vi "Host.vi"() -> ()   [LabVIEW 2017]
uses:
  <vilib>/NI/STM/TCP/TCP Read Options.ctl
  TypeDefs/Data for Logging.ctl
  TypeDefs/ClientStatusData.ctl
  <vilib>/NI/STM/TCP/Read Meta Data (TCP Ref).vi
  <vilib>/NI/STM/TCP/Get Connection Reference (TCP).vi
  <vilib>/NI/STM/TCP/Read Meta Data (TCP Clst).vi
  <vilib>/NI/STM/TCP/Write Message (TCP).vi
  <vilib>/NI/STM/TCP/Read Message (TCP).vi
  <vilib>/NI/STM/NI STM.lvlib
panel:
  out "Numeric 2":dbl
  out "Numeric":dbl
  in  "C":dbl=1.0
  in  "K":dbl=1.0
  in  "D":dbl
  in  "I":dbl
  in  "P":dbl=0.2
  in  "Update":bool
  in  "testingtargetY":dbl=0.1
  in  "testingtargetX":dbl=0.1
  in  "Testing?":bool
  out "RECENT PLAYERS":string[](array[string])
  out "X POSITION":cluster{dbl, dbl}(graph)
  out "Y POSITION":cluster{dbl, dbl}(graph)
  out "?":cluster{dbl[], dbl[]}[](graph)
  in  "assistance":bool
  out "error  out":errorcluster
  in  "stop":bool
  # "zero gains here create NaN (bad for controller)"
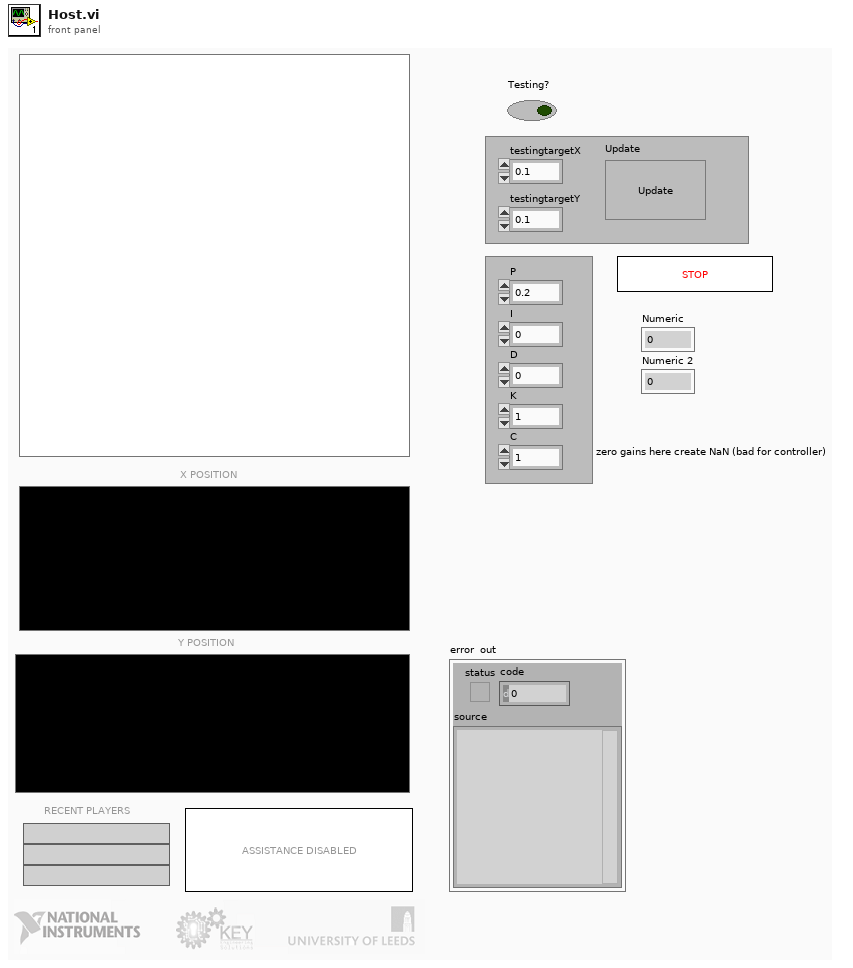
[diagram p1: front panel]
types:
  T1 = typedef "NI STM.lvlib/TCP Connection Info.ctl" = cluster{"connection ID":refnum<k5>, "meta data":T2[]}
  T2 = typedef "NI STM.lvlib/MetaDataElement.ctl" = string
  T3 = typedef "NI STM.lvlib/TCP Read Options.ctl" = cluster{"ignore timeout error":bool, "timeout ms (1000)":i32}
  T4 = enum16{"open", "replace", "create", "open or create", "replace or create", "replace or create with confirmation"}
  T5 = typedef "Data for Logging.ctl" = cluster{"end effector x (mm)":dbl, "end effector y (mm)":dbl, "target x (mm)":dbl, "target y (mm)":dbl, "Theta 1":dbl, "Theta 2":dbl, "Omega 1":dbl, "Omega 2":dbl}
  T6 = typedef "ClientStatusData.ctl" = cluster{"gameState":u16, "playerName":string, "playerScore":dbl, "gameUnits":string}
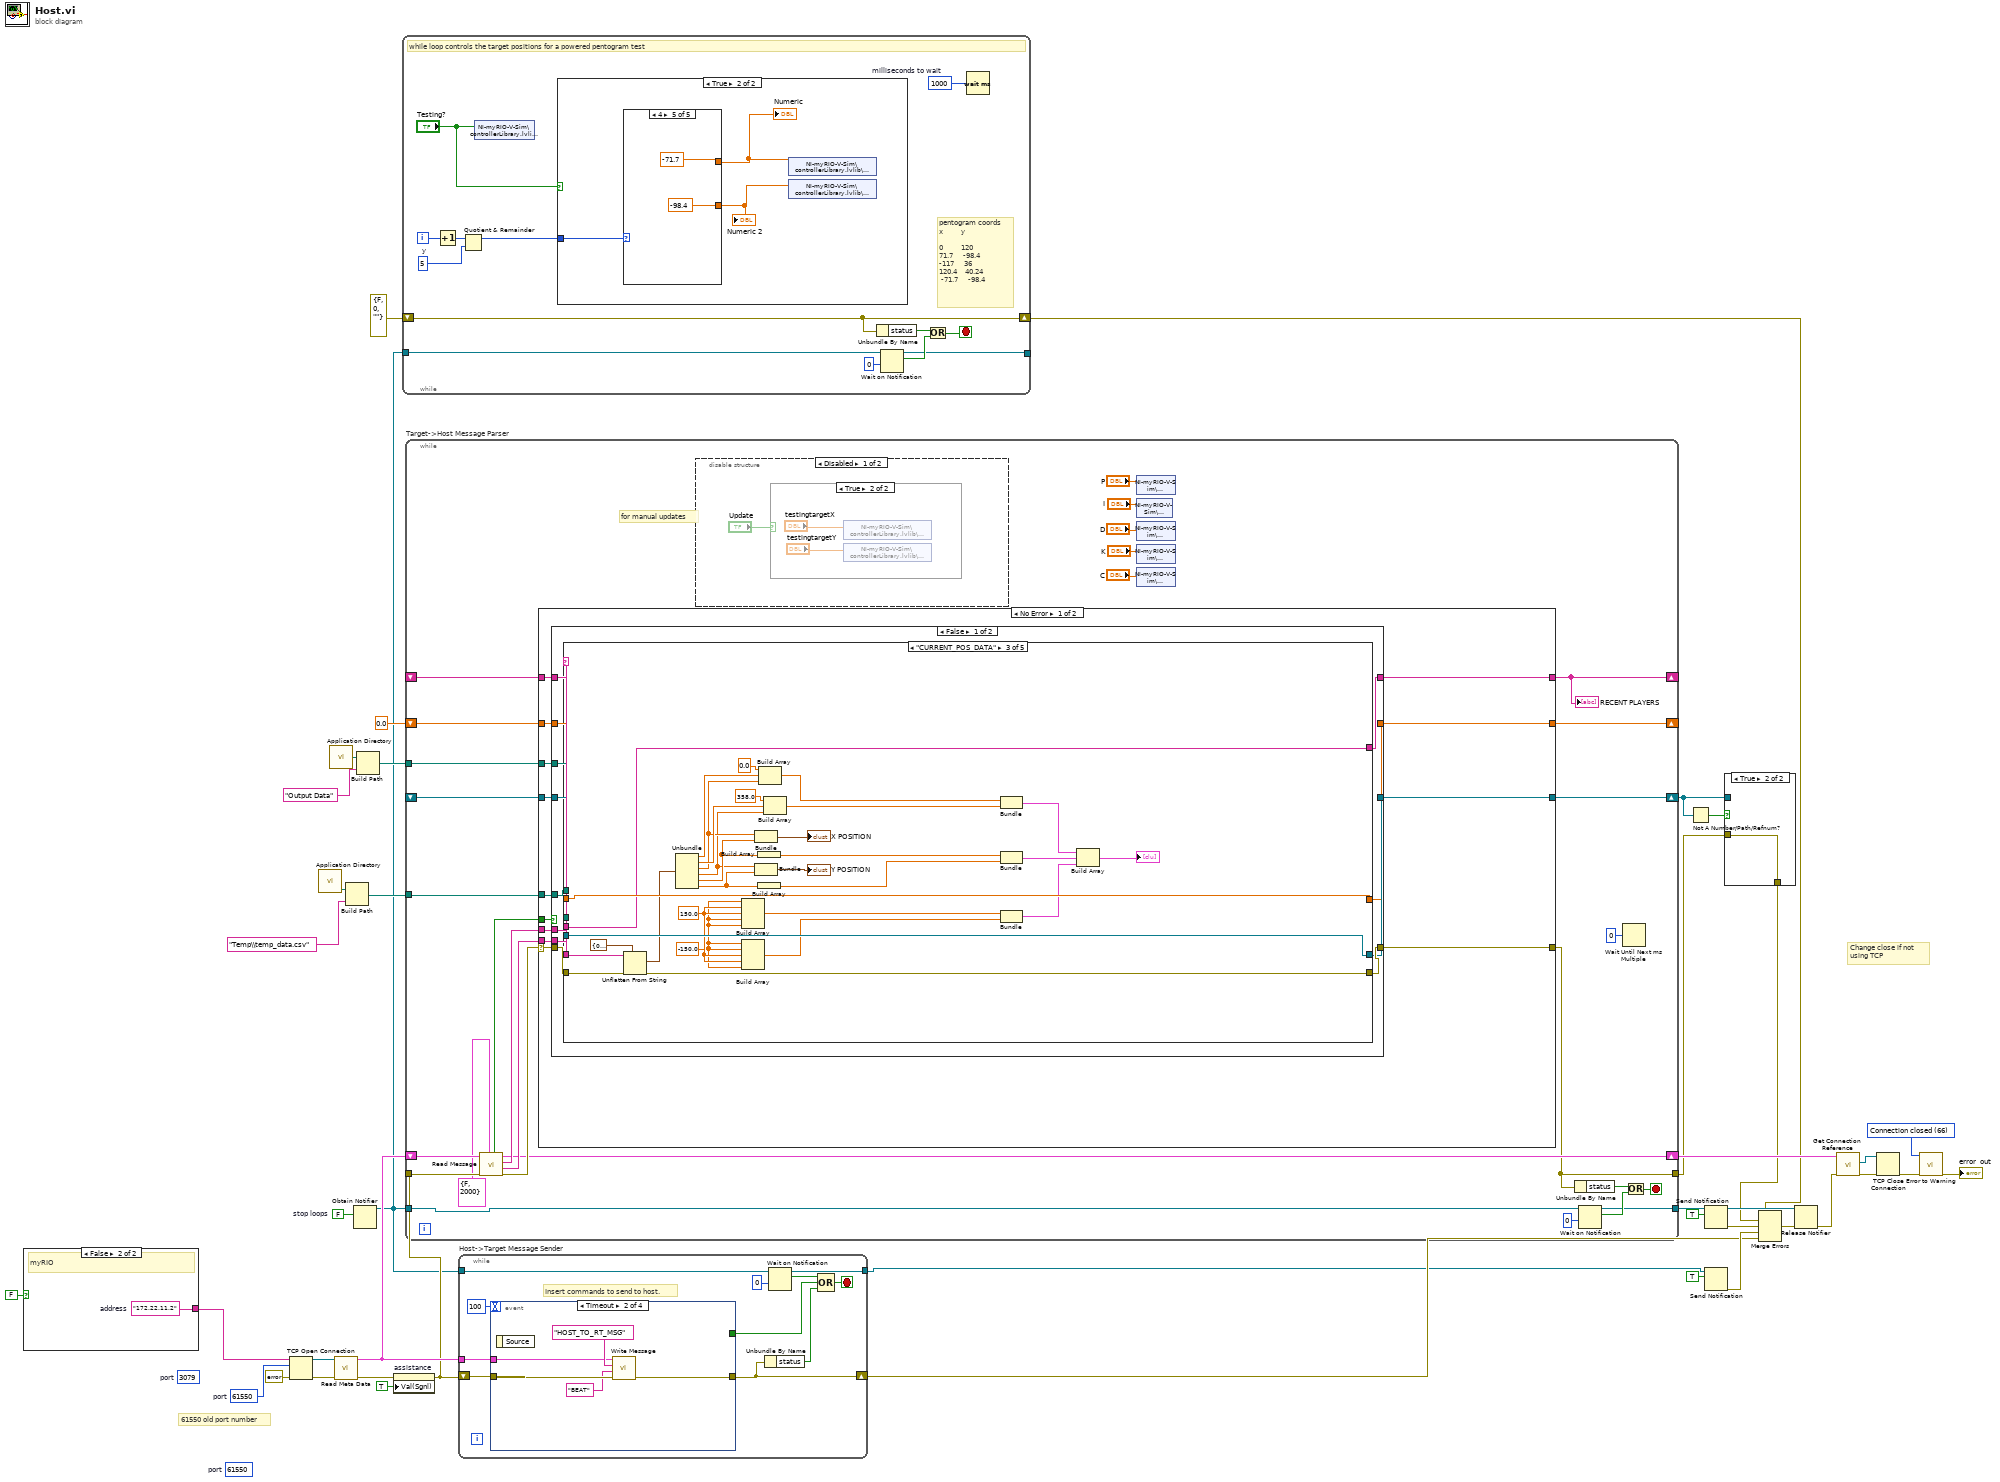
[diagram p0: block diagram]
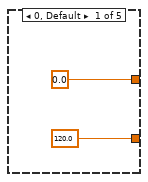
[diagram p3: hidden frame]
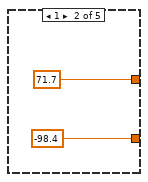
[diagram p4: hidden frame]
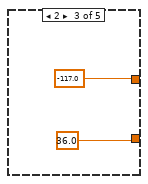
[diagram p5: hidden frame]
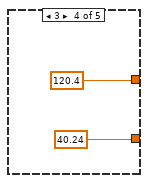
[diagram p6: hidden frame]
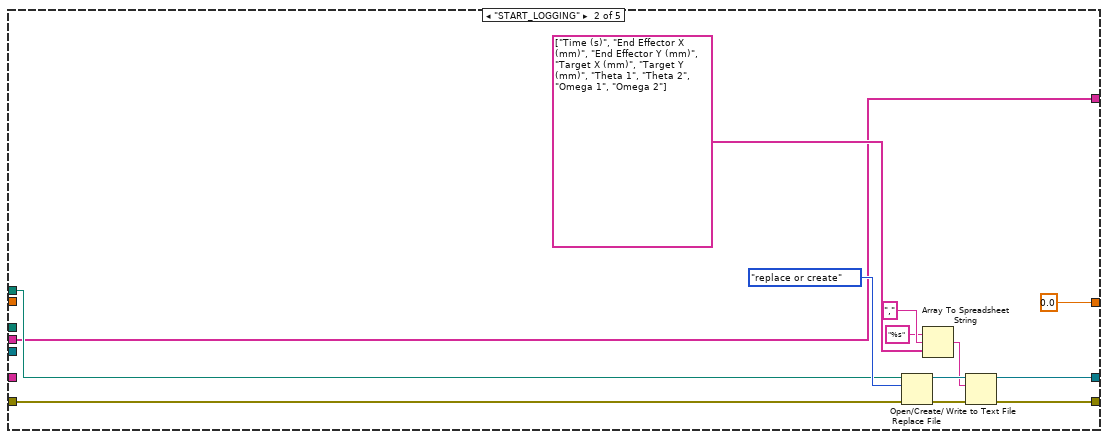
[diagram p10: hidden frame]
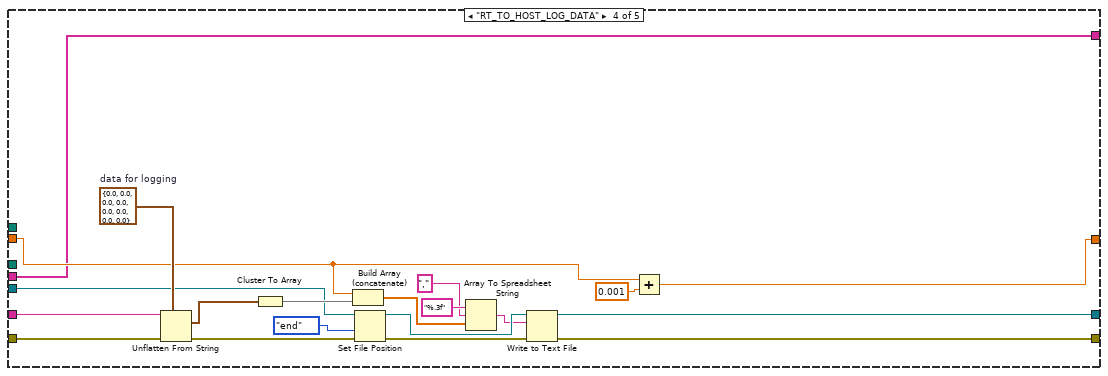
[diagram p11: hidden frame]
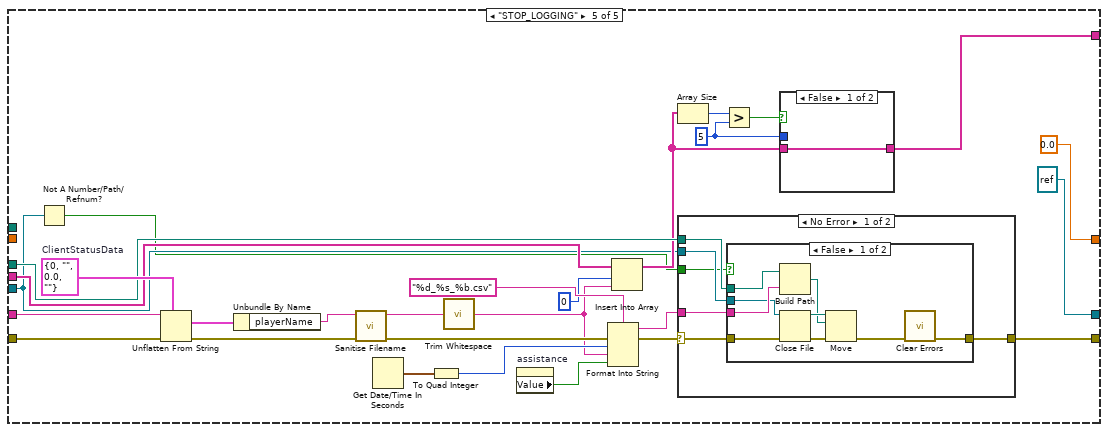
[diagram p12: hidden frame]
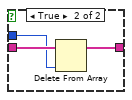
[diagram p15: hidden frame]
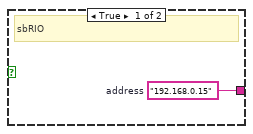
[diagram p18: hidden frame]
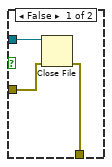
[diagram p19: hidden frame]
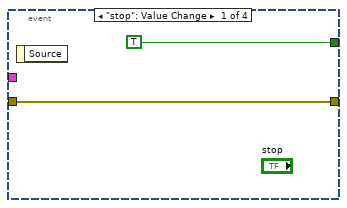
[diagram p20: hidden frame]
diagram:
  (unwired) u16 61550  # port
  w5 = u16 61550  # port
  w26 = FALSE  # stop loops
  w37 = 66 items=["No Error", "Argument Error", "Memory Full", "Out of Zone", "End of File", "File Already Open", "Generic File IO Error", "File Not Found", "File Permission Error", "Disk Full", "Duplicate Path", "Too Many Files Open", "Not Enabled", "Resource File Not Found", "Cannot Add Resource", "Resource Not Found", "Image Not Found", "Image Memory Error", "Pen Does Not Exist", "Config Bad Type", "Config Token Not Found", "Config Parse Error", "Config Memory Error", "Bad External Code Format", "Bad External Code Offset", "External Code Not Present", "Null Window", "Destroy Window Mixup", "Null Menu", "Print Aborted", "Bad Print Record", "Print Driver Error", "Windows Error During Print", "Memory Error During Print", "Print Dialog Error", "Generic Print Error", "Invalid Device Refnum", "Device Not Found", "Device Parameter Error", "Device Unit Error", "Can't Open Device", "Device Call Aborted", "Generic Error", "Cancelled By User", "Object ID Too Low", "Object ID Too High", "Object Not In Heap", "Unknown Heap", "Bad DefProc ID", "DefProc Not In Table", "Message Out Of Range", "Null Method", "Unknown Message", "Manager Call Not Supported", "Bad address", "Connection In progress", "Connection timed out", "Connection is already in progress", "Network attribute not supported", "Network error", "Address in use", "System out of memory", "Connection aborted", "Connection refused", "Connection is not connected", "Connection is already connected", "Connection closed", "Initialize error (interapplication manager)", "Bad occurrence", "Wait on unbound occurrence handler", "Occurrence queue overflow", "Bad path", "Semaphore not signaled", "Unrecognized type (interapplication manager)"] ("1st Error to Convert")
  (unwired) u16 3079  # port
  # "61550 old port number"
  # "Change close if not using TCP"
  n1 = case shown="False" FALSE {
    tunnel: [w42 w43] -> w41
    frame True {
      w42 = "192.168.0.15"  # address
      # "sbRIO"
    }
    frame False {
      w43 = "172.22.11.2"  # address
      # "myRIO"
    }
  }
  n2 = TCP Open Connection(address=w41, remote port or service name=w5, error in (no error)=errorcluster {"status"=FALSE, "code"=0, "source"=""}) -> (connection ID=w21:refnum<k5>, error out=w20:errorcluster)  [unwired: 2 in]
  n3 = call <vilib>:"Application Directory.vi"() -> ("Application Directory"=w18:path)
  n4 = call <vilib>:"Application Directory.vi"() -> ("Application Directory"=w16:path)
  n5 = call-poly <vilib>:"Read Meta Data.vi"("error in"=w20, "connection ID"=w21) -> ("error out"=w11:errorcluster, "connection info out"=w24:T1)  [unwired: 1 in, 7 out]
  n6 = Build Path(base path=w18, name or relative path="Temp\\temp_data.csv") -> (appended path=w17:path)
  n7 = Obtain Notifier(notification data type=w26) -> (notifier out=w3:refnum<notifier>)  [unwired: 3 in, 2 out]
  n8 = Build Path(base path=w16, name or relative path="Output Data") -> (appended path=w14:path)
  n9 = property on="assistance" class="Bool (strict)"(error in=w11, "Val(Sgnl)"=TRUE ("Value (Signaling)")) -> (error out=w10:errorcluster)  [unwired: 1 in, 1 out]
  n10 = while {
    tunnel: w3 -> [w53]
    tunnel: [w52] -> _
    shift-right: [w50] -> w1
    shift-left: errorcluster {"status"=FALSE, "code"=0, "source"=""} ("error constant") -> [w50]
    i -> [w47]
    stop <- w51 stop-if-true
    w45 = 5  # y
    w48 = u32 1000  # milliseconds to wait
    # "pentogram coords\nx         y \n\n0         120\n71.7     -98.4\n-117     36\n120.4    40.24 \n -71.7     -98.4"
    # "while loop controls the target positions for a powered pentogram test"
    n11 = Increment(x=w47) -> (x+1=w46:i32)
    n12 = Quotient & Remainder(x=w46, y=w45) -> (x-y*floor(x/y)=w44:i32)  [unwired: 1 out]
    n13 = shared-variable "NI-myRIO-V-Sim\\controllerLibrary.lvlib\\testing"("Testing?") -> ()  [unwired: 1 in, 1 out]
    n14 = case shown="True" "Testing?" {
      tunnel: w44 -> [_ w59]
      frame False {
      }
      frame True {
        n15 = case shown="4" w59 {
          tunnel: [0.0 71.7 -117.0 120.4 -71.7] -> w58
          tunnel: [120.0 -98.4 36.0 40.24 -98.4] -> w57
          frame 0, Default {
          }
          frame 1 {
          }
          frame 2 {
          }
          frame 3 {
          }
          frame 4 {
          }
        }
        "Numeric" <- w58
        "Numeric 2" <- w57
        n16 = shared-variable "NI-myRIO-V-Sim\\controllerLibrary.lvlib\\testingtargetX"(w58) -> ()  [unwired: 1 in, 1 out]
        n17 = shared-variable "NI-myRIO-V-Sim\\controllerLibrary.lvlib\\testingtargetY"(w57) -> ()  [unwired: 1 in, 1 out]
      }
    }
    n18 = Unbundle By Name(w50) -> ("status"=w54:bool)
    n19 = Wait on Notification(notifier=w53, timeout in ms (-1)=0) -> (notifier out=w52:refnum<notifier>, notification=w55:bool)  [unwired: 2 in, 2 out]
    n20 = Or(x=w54, y=w55) -> (x .or. y?=w51:bool)
    n21 = Wait (ms)(milliseconds to wait=w48) -> ()  [unwired: 1 out]
  }
  n22 = while "Target->Host Message Parser" {
    tunnel: w3 -> [w91]
    tunnel: [w87] -> w27
    shift-right: [w92] -> w25
    shift-left: w24 -> [w98]
    tunnel: w17 -> [w83]
    tunnel: w14 -> [w82]
    shift-right: [w81] -> w8
    shift-left: _ -> [w80]
    shift-right: [w78] -> _
    shift-left: 0.0 -> [w79]
    shift-right: [w76] -> _
    shift-left: _ -> [w77]
    tunnel: w10 -> [w97]
    tunnel: [w85] -> w4
    stop <- w88 stop-if-true
    # "for manual updates"
    n23 = call-poly <vilib>:"Read Message.vi"("options"=T3 {"ignore timeout error"=FALSE, "timeout ms (1000)"=2000}, "error in"=w97, "connection info in"=w98) -> ("error out"=w93:errorcluster, "name"=w96:T2, "data string"=w95:string, "connection info out"=w92:T1, "timed out?"=w94:bool)  [unwired: 2 in, 2 out]
    n24 = case shown="No Error" w93 {
      selector: w93 -> [w111 w250]
      tunnel: w96 -> [w114 _]
      tunnel: w95 -> [w113 _]
      tunnel: w94 -> [w112 _]
      tunnel: [w110 w250] -> w85
      tunnel: w83 -> [w109 _]
      tunnel: w82 -> [w108 _]
      tunnel: [w107 w249] -> w81
      tunnel: w80 -> [w106 w249]
      tunnel: w79 -> [w105 w248]
      tunnel: [w104 w248] -> w78
      tunnel: w77 -> [w103 w247]
      tunnel: [w102 w247] -> w76
      frame No Error {
        n25 = case shown="False" w112 {
          tunnel: w114 -> [w123 _]
          tunnel: w113 -> [w126 _]
          tunnel: w111 -> [w125 w246]
          tunnel: [w124 w246] -> w110
          tunnel: w109 -> [w122 _]
          tunnel: w108 -> [w121 _]
          tunnel: [w120 w245] -> w107
          tunnel: w106 -> [w119 w245]
          tunnel: w105 -> [w118 w244]
          tunnel: [w117 w244] -> w104
          tunnel: w103 -> [w116 w243]
          tunnel: [w115 w243] -> w102
          frame False {
            n26 = case shown="\"CURRENT_POS_DATA\"" w123 {
              tunnel: w126 -> [_ _ w170 w191 w219]
              tunnel: w125 -> [w128 w142 w169 w193 w221]
              tunnel: [w128 w139 w168 w177 w195] -> w124
              tunnel: w122 -> [_ w141 _ _ _]
              tunnel: w121 -> [_ _ _ _ w213]
              tunnel: [w130 w138 w172 w176 refnum<file> refnum ("refnum out")] -> w120
              tunnel: w119 -> [w130 _ w172 w175 w197]
              tunnel: w118 -> [w129 _ w173 w186 _]
              tunnel: [w129 0.0 w173 w188 0.0] -> w117
              tunnel: w116 -> [w127 w131 w147 w174 w205]
              tunnel: [w127 w131 w147 w174 w200] -> w115
              frame Default {
              }
              frame "START_LOGGING" {
                n27 = Open/Create/Replace File(file path (use dialog)=w141, error in=w142, operation (0:open)=T4."replace or create") -> (refnum out=w134:refnum<file>, error out=w135:errorcluster)  [unwired: 3 in, 1 out]
                n28 = Array To Spreadsheet String(delimiter (Tab)=",", array=string[] ["Time (s)", "End Effector X (mm)", "End Effector Y (mm)", "Target X (mm)", "Target Y (mm)", "Theta 1", "Theta 2", "Omega 1", "Omega 2"], 3:"%s" ("format string")) -> (spreadsheet string=w133:string)
                n29 = Write to Text File(file (use dialog)=w134, text=w133, error in=w135) -> (refnum out=w138:refnum<file>, error out=w139:errorcluster)  [unwired: 1 in, 1 out]
              }
              frame "CURRENT_POS_DATA" {
                w152 = -150.0
                w153 = 150.0
                n30 = Unflatten From String(type=cluster{dbl, dbl, dbl, dbl, dbl, dbl} {0.0, 0.0, 0.0, 0.0, 0.0, 0.0}, binary string=w170, error in (no error)=w169) -> (value=w167:cluster{dbl, dbl, dbl, dbl, dbl, dbl}, error out=w168:errorcluster)  [unwired: 2 in, 1 out]
                n31 = Unbundle(w167) -> (w164:dbl, w163:dbl, w145:dbl, w144:dbl, w150:dbl, w151:dbl)
                n32 = Build Array(w152, w153, w153, w152, w152) -> (w155:dbl[])
                n33 = Build Array(w152, w152, w153, w153, w152) -> (w154:dbl[])
                n34 = Bundle(w145, w150) -> (→"X POSITION":cluster{dbl, dbl})  [unwired: 1 in]
                n35 = Bundle(w144, w151) -> (→"Y POSITION":cluster{dbl, dbl})  [unwired: 1 in]
                n36 = Build Array(w150) -> (w158:dbl[])
                n37 = Build Array(w151) -> (w157:dbl[])
                n38 = Build Array(0.0 ("element"), w164, w145) -> (w162:dbl[])
                n39 = Build Array(358.0 ("element"), w163, w144) -> (w161:dbl[])
                n40 = Bundle(w162, w161) -> (w160:cluster{dbl[], dbl[]})  [unwired: 1 in]
                n41 = Bundle(w158, w157) -> (w156:cluster{dbl[], dbl[]})  [unwired: 1 in]
                n42 = Bundle(w155, w154) -> (w146:cluster{dbl[], dbl[]})  [unwired: 1 in]
                n43 = Build Array(w160, w156, w146) -> (→"?":cluster{dbl[], dbl[]}[])
              }
              frame "RT_TO_HOST_LOG_DATA" {
                w192 = T5 {"end effector x (mm)"=0.0, "end effector y (mm)"=0.0, "target x (mm)"=0.0, "target y (mm)"=0.0, "Theta 1"=0.0, "Theta 2"=0.0, "Omega 1"=0.0, "Omega 2"=0.0}  # data for logging
                n44 = Unflatten From String(type=w192, binary string=w191, error in (no error)=w193) -> (value=w190:T5, error out=w182:errorcluster)  [unwired: 2 in, 1 out]
                n45 = Cluster To Array(cluster=w190) -> (array=w187:dbl[])
                n46 = Build Array (concatenate)(w186, w187) -> (w185:dbl[])
                n47 = Set File Position(refnum=w175, from (0:start)=enum16{"start", "end", "current"}."end", error in=w182) -> (refnum out=w179:refnum<file>, error out=w180:errorcluster)  [unwired: 1 in]
                n48 = Array To Spreadsheet String(delimiter (Tab)=",", array=w185, 3:"%.3f" ("format string")) -> (spreadsheet string=w178:string)
                n49 = Write to Text File(file (use dialog)=w179, text=w178, error in=w180) -> (refnum out=w176:refnum<file>, error out=w177:errorcluster)  [unwired: 1 in, 1 out]
                n50 = Add(x=w186, y=0.001) -> (x+y=w188:dbl)
              }
              frame "STOP_LOGGING" {
                w201 = 5 ("y")
                w220 = T6 {"gameState"=0, "playerName"="", "playerScore"=0.0, "gameUnits"=""}  # ClientStatusData
                n51 = Not A Number/Path/Refnum?(number/path/refnum=w197) -> (NaN/Path/Refnum?=w196:bool)
                n52 = Unflatten From String(type=w220, binary string=w219, error in (no error)=w221) -> (value=w217:T6, error out=w209:errorcluster)  [unwired: 2 in, 1 out]
                n53 = Unbundle By Name(w217) -> ("playerName"=w207:string)
                n54 = call "Sanitise Filename.vi"("error in"=w209, "input filename"=w207) -> ("error out"=w208:errorcluster, "output filename"=w206:string)  [unwired: 8 in]
                n55 = Get Date/Time In Seconds() -> (seconds since 1Jan1904=w216:timestamp)
                n56 = To Quad Integer(1:w216) -> (0:w215:i64)
                n57 = call <vilib>:"Trim Whitespace.vi"("string"=w206) -> ("trimmed string"=w199:string)  [unwired: 1 in]
                n58 = property on="assistance" class="Bool (strict)"() -> ("Value"=w194:bool)  [unwired: 2 in, 2 out]
                n59 = Format Into String(format string="%d_%s_%b.csv", error in=w208, w215, w199, w194) -> (resulting string=w212:string, error out=w210:errorcluster)  [unwired: 1 in]
                n60 = Insert Into Array(array=w205, index=0, new element=w199) -> (w202:string[])
                n61 = Array Size(array=w202) -> (size(s)=w204:i32)
                n62 = case shown="No Error" w210 {
                  selector: w210 -> [w225 w238]
                  tunnel: w213 -> [w227 _]
                  tunnel: w212 -> [w226 _]
                  tunnel: w197 -> [w224 _]
                  tunnel: w196 -> [w223 _]
                  tunnel: [w222 w238] -> w195
                  frame No Error {
                    n63 = case shown="False" w223 {
                      tunnel: w227 -> [w236 _]
                      tunnel: w226 -> [w235 _]
                      tunnel: w225 -> [w232 w237]
                      tunnel: w224 -> [w230 _]
                      tunnel: [w228 w237] -> w222
                      frame False {
                        n64 = Build Path(base path=w236, name or relative path=w235) -> (appended path=w233:path)
                        n65 = Close File(refnum=w230, error in=w232) -> (path=w234:path, error out=w231:errorcluster)
                        n66 = Move(source path=w234, error in=w231, 10:w233) -> (error out=w229:errorcluster)  [unwired: 2 in, 2 out]
                        n67 = call <vilib>:"Clear Errors.vi"("error in (no error)"=w229) -> ("error out"=w228:errorcluster)  [unwired: 5 in, 1 out]
                      }
                      frame True {
                      }
                    }
                  }
                  frame Error {
                  }
                }
                n68 = Greater?(x=w204, y=w201) -> (0:w203:bool)
                n69 = case shown="False" w203 {
                  tunnel: w202 -> [w239 w242]
                  tunnel: w201 -> [_ w241]
                  tunnel: [w239 w240] -> w200
                  frame False {
                  }
                  frame True {
                    n70 = Delete From Array(array=w242, index=w241) -> (array with subset deleted=w240:string[])  [unwired: 1 in, 1 out]
                  }
                }
              }
            }
          }
          frame True {
          }
        }
      }
      frame Error {
      }
    }
    "RECENT PLAYERS" <- w76
    n71 = disable-structure shown="Disabled" {
      frame Disabled {
        n72 = case shown="True" "Update" {
          frame False {
          }
          frame True {
            n73 = shared-variable "NI-myRIO-V-Sim\\controllerLibrary.lvlib\\testingtargetX"("testingtargetX") -> ()  [unwired: 1 in, 1 out]
            n74 = shared-variable "NI-myRIO-V-Sim\\controllerLibrary.lvlib\\testingtargetY"("testingtargetY") -> ()  [unwired: 1 in, 1 out]
          }
        }
      }
      frame Enabled {
      }
    }
    n75 = shared-variable "NI-myRIO-V-Sim\\controllerLibrary.lvlib\\P"("P") -> ()  [unwired: 1 in, 1 out]
    n76 = shared-variable "NI-myRIO-V-Sim\\controllerLibrary.lvlib\\I"("I") -> ()  [unwired: 1 in, 1 out]
    n77 = shared-variable "NI-myRIO-V-Sim\\controllerLibrary.lvlib\\D"("D") -> ()  [unwired: 1 in, 1 out]
    n78 = shared-variable "NI-myRIO-V-Sim\\controllerLibrary.lvlib\\K"("K") -> ()  [unwired: 1 in, 1 out]
    n79 = shared-variable "NI-myRIO-V-Sim\\controllerLibrary.lvlib\\C"("C") -> ()  [unwired: 1 in, 1 out]
    n80 = Unbundle By Name(w85) -> ("status"=w86:bool)
    n81 = Wait on Notification(notifier=w91, timeout in ms (-1)=0) -> (notifier out=w87:refnum<notifier>, notification=w89:bool)  [unwired: 2 in, 2 out]
    n82 = Wait Until Next ms Multiple(millisecond multiple=u32 0) -> ()  [unwired: 1 out]
    n83 = Or(x=w86, y=w89) -> (x .or. y?=w88:bool)
  }
  n84 = while "Host->Target Message Sender" {
    shift-right: [w253] -> w31
    shift-left: w10 -> [w261]
    tunnel: w24 -> [w260]
    tunnel: w3 -> [w257]
    tunnel: [w254] -> w29
    stop <- w255 stop-if-true
    # "Insert commands to send to host."
    n85 = event shown="[1] Timeout" {
      selector: _ -> [_ _ _ _]
      dyn-events: _ -> [_ _ _ _]
      timeout: 100 -> [_ _ _ _]
      tunnel: w260 -> [_ w265 w273 _]
      tunnel: w261 -> [w263 w268 w276 w277]
      tunnel: [TRUE ("stop") _ _ TRUE ("stop")] -> w252
      tunnel: [w263 w267 w275 w277] -> w253
      event "stop": Value Change {
        n86 = event-data() -> ()  [unwired: 2 out]
      }
      event Timeout {
        n87 = event-data() -> ()  [unwired: 2 out]
        n88 = call-poly <vilib>:"Write Message.vi"("error in"=w268, "data"="BEAT", "name"="HOST_TO_RT_MSG", "connection info in"=w265) -> ("error out"=w267:errorcluster)  [unwired: 1 in, 6 out]
      }
      event "assistance": Value Change {
        n89 = event-data() -> ()  [unwired: 2 out]
        n90 = Select(t="ENABLE_ASSISTANCE" ("data"), s="assistance", f="DISABLE_ASSISTANCE" ("data")) -> (s? t:f=w269:string)
        n91 = call-poly <vilib>:"Write Message.vi"("error in"=w276, "data"=w269, "name"="HOST_TO_RT_MSG", "connection info in"=w273) -> ("error out"=w275:errorcluster)  [unwired: 1 in, 6 out]
      }
      event Panel Close? {
        n92 = event-data() -> ()  [unwired: 5 out]
        n93 = event-data("Discard?"=TRUE) -> ()  [unwired: 1 in, 1 out]
      }
    }
    n94 = Unbundle By Name(w253) -> ("status"=w251:bool)
    n95 = Wait on Notification(notifier=w257, timeout in ms (-1)=0) -> (notifier out=w254:refnum<notifier>, notification=w259:bool)  [unwired: 2 in, 2 out]
    n96 = Compound Arithmetic op=OR(w259, w252, w251) -> (w255:bool)
  }
  n97 = Not A Number/Path/Refnum?(number/path/refnum=w8) -> (NaN/Path/Refnum?=w9:bool)
  n98 = Send Notification(notification=TRUE, notifier=w27) -> (notifier out=w34:refnum<notifier>, error out=w33:errorcluster)  [unwired: 1 in]
  n99 = Send Notification(notification=TRUE, notifier=w29) -> (error out=w32:errorcluster)  [unwired: 1 in, 1 out]
  n100 = case shown="True" w9 {
    tunnel: w8 -> [w282 _]
    tunnel: w4 -> [w281 w283]
    tunnel: [w280 w283] -> w7
    frame False {
      n101 = Close File(refnum=w282, error in=w281) -> (error out=w280:errorcluster)  [unwired: 1 out]
    }
    frame True {
    }
  }
  n102 = Merge Errors(w1, w7, w33, w32, w31) -> (w35:errorcluster)
  n103 = Release Notifier(notifier=w34, error in (no error)=w35) -> (error out=w36:errorcluster)  [unwired: 1 in, 2 out]
  n104 = call-poly <vilib>:"Get Connection Reference.vi"("error in"=w36, "connection info in"=w25) -> ("error out"=w23:errorcluster, "connection ID out"=w22:refnum<k5>)  [unwired: 8 out]
  n105 = TCP Close Connection(connection ID=w22, error in (no error)=w23) -> (error out=w38:errorcluster)  [unwired: 2 out]
  n106 = call <vilib>:"Error to Warning.vi"("1st Error to Convert"=w37, "error in"=w38) -> ("warning out"=→"error  out":errorcluster)  [unwired: 3 in, 10 out]
